vi "sumOfFrequencies.vi"(6 "frequency":dbl, 9 "signal type":enum16{"Sine", "Square", "Sawtooth", "Random"}(ring), 10 "offset":dbl, 11 "amplitude":dbl) -> (3 "Numeric":dbl)   [LabVIEW 2020]
uses:
  <vilib>/Simulation/Implementation/Shared/SIMSCR Execution Mode.ctl
  <vilib>/Simulation/Scripting/Companion Diagram/SimConfigNode/SimParams.ctl
  <vilib>/Simulation/Scripting/Companion Diagram/SimConfigNode/_simSolvers.ctl
  <vilib>/Simulation/Param Hierarchy/Typedefs/SIMPH Param Control Actions.ctl
  <vilib>/Simulation/Implementation/Shared/NILVSim_ParamChanged.vi
  <vilib>/Simulation/Implementation/Shared/NILVSIM_BeginStep.vi
  <vilib>/Simulation/DataSources/Implementation/NILVSim Signal Generator.llb/SIM Signal Generator (scalar).vi
  <vilib>/Simulation/Implementation/Shared/NILVSim_Manager.vi
  <vilib>/Utility/error.llb/Clear Errors.vi
  <vilib>/Simulation/Implementation/Shared/NILVSim_FinalizeModel.vi
  <vilib>/Simulation/Implementation/Shared/SIM Unbundle Sim Info.vi
  <vilib>/Simulation/Implementation/Shared/NILVSim_Initialize.vi
  <vilib>/Simulation/Utility/Implementation/NILVSim Get Time and IsAcceptedStep.vi
  <vilib>/Simulation/Implementation/Shared/NILVSim_GetModelError.vi
  <vilib>/Simulation/Implementation/Shared/SIM SimErrorHandler.vi
  <vilib>/Simulation/Implementation/Shared/SIMSH Read Queue.vi
  <vilib>/Simulation/Implementation/Shared/SIM Bundle Sim Info.vi
  <vilib>/Simulation/Scripting/Companion Diagram/SimConfigNode/SimDog.xnode
  <vilib>/Simulation/Implementation/XNodeFramework/SimXNode/SimX.xnode
  <vilib>/Simulation/Implementation/Shared/NI_SIM_Implementation.lvlib
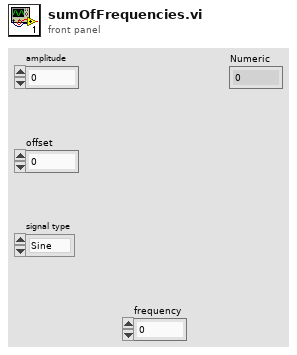
[diagram p1: front panel]
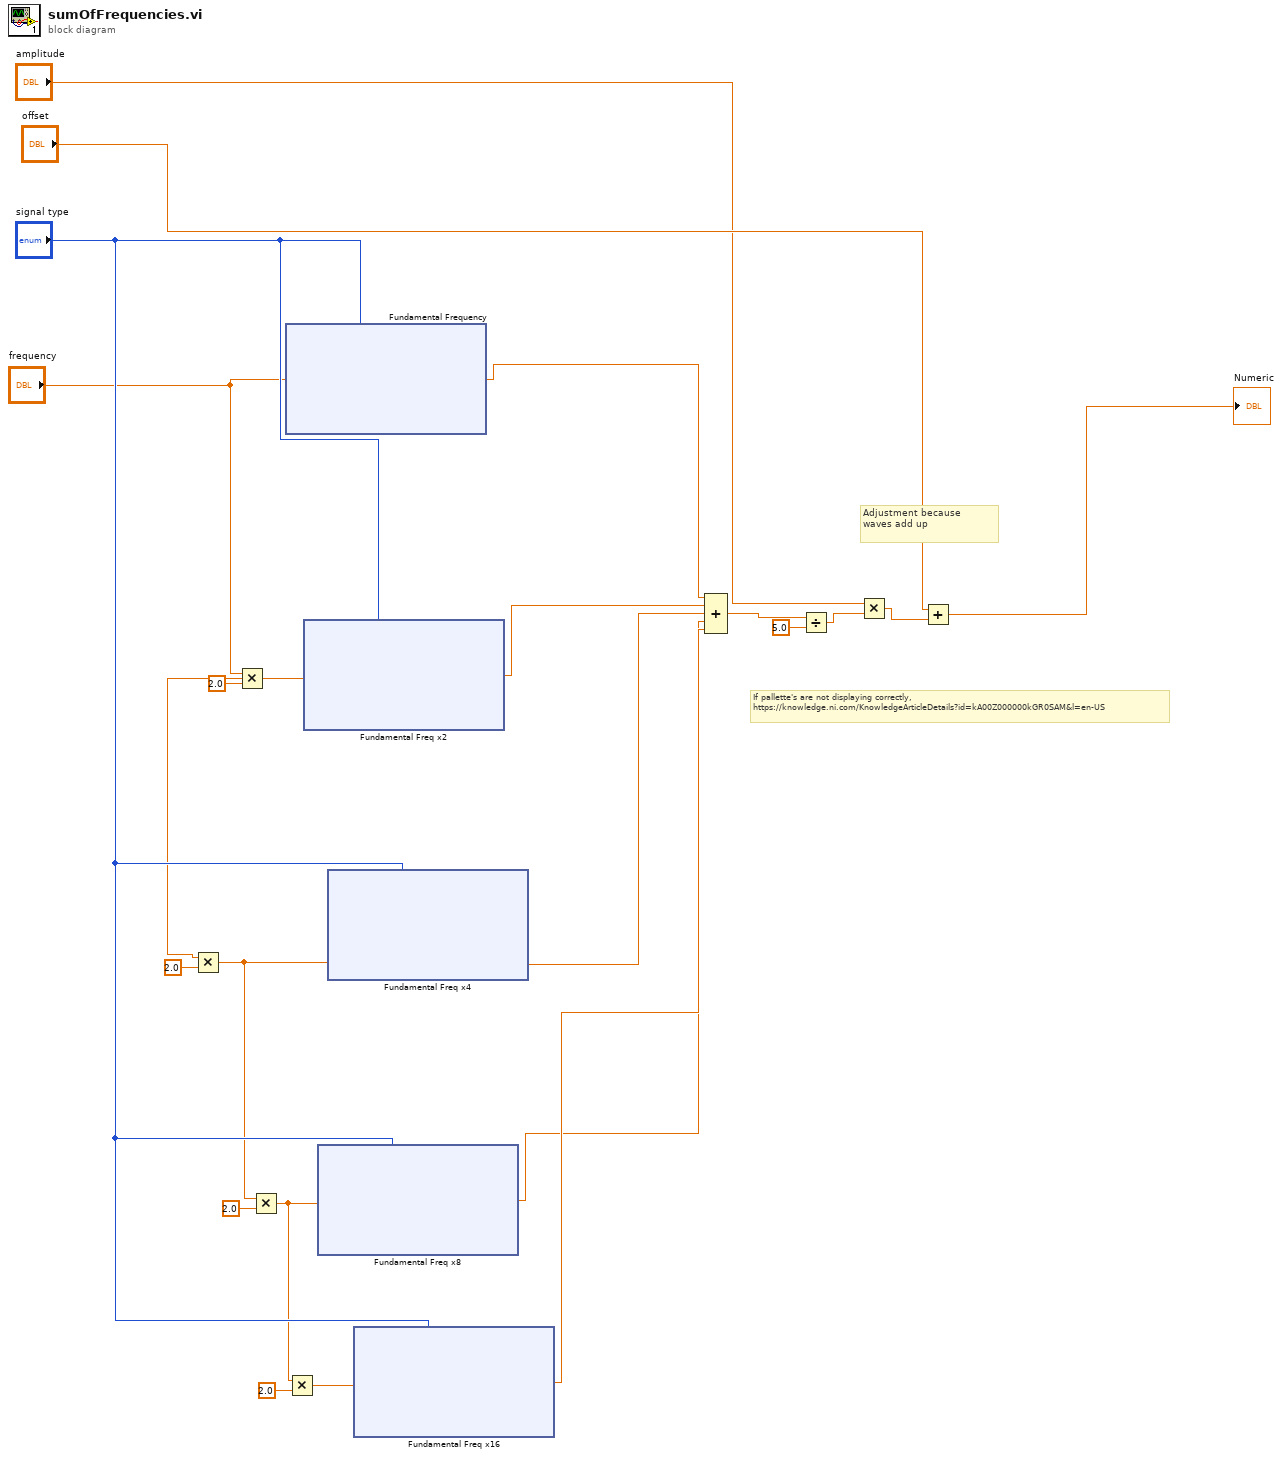
[diagram p0: block diagram]
diagram:
  # "Adjustment because \nwaves add up"
  # "If pallette's are not displaying correctly,\nhttps://knowledge.ni.com/KnowledgeArticleDetails?id=kA00Z000000kGR0SAM&l=en-US"
  n1 = Multiply(x="frequency", y=2.0) -> (x*y=w6:dbl)
  n2 = Multiply ("Multiply 2")(x=w6, y=2.0 ("y 2")) -> (x*y=w10:dbl)
  n3 = Multiply ("Multiply 3")(x=w10, y=2.0 ("y 3")) -> (x*y=w14:dbl)
  n4 = xnode "Fundamental Frequency"("signal type"="signal type", "frequency"="frequency") -> ("output"=w2:dbl)  [unwired: 5 in]
  n5 = Multiply ("Multiply 4")(x=w14, y=2.0 ("y 4")) -> (x*y=w12:dbl)
  n6 = xnode "Fundamental Freq x2"("signal type"="signal type", "frequency"=w6) -> ("output"=w1:dbl)  [unwired: 5 in]
  n7 = xnode "Fundamental Freq x8"("signal type"="signal type", "frequency"=w14) -> ("output"=w9:dbl)  [unwired: 5 in]
  n8 = xnode "Fundamental Freq x4"("signal type"="signal type", "frequency"=w10) -> ("output"=w7:dbl)  [unwired: 5 in]
  n9 = xnode "Fundamental Freq x16"("signal type"="signal type", "frequency"=w12) -> ("output"=w13:dbl)  [unwired: 5 in]
  n10 = Compound Arithmetic op=ADD(w2, w1, w7, w9, w13) -> (w16:dbl)
  n11 = Divide(x=w16, y=5.0 ("y 5")) -> (x/y=w18:dbl)
  n12 = Multiply ("Multiply 5")(x="amplitude", y=w18) -> (x*y=w20:dbl)
  n13 = Add(x="offset", y=w20) -> (x+y=→"Numeric":dbl)
